vi "Get Index and Type.vi"(8 "error in (no error)":errorcluster, 11 "Tag":string) -> (0 "error out":errorcluster, 2 "Type":T1, 3 "Index":i32)   [LabVIEW 2016, in "CVT.lvlib" / "Current Value Table.lvlib"]
doc: "This VI retrieves a group of indices as defined by the tag names provided. These tags must be retrieved as a single type. If multiple types are requested, error 537165 will be thrown."
uses:
  <vilib>/NI/Current Value Table/Current Value Table.lvlib
  <vilib>/NI/Current Value Table/Type Defs/Data Types.ctl
  <vilib>/NI/Current Value Table/FGVs/Tag Memory Methods.ctl
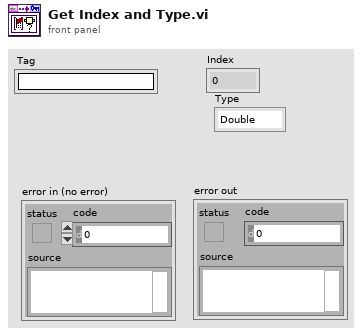
[diagram p1: front panel]
types:
  T1 = typedef "CVT.lvlib/Current Value Table.lvlib/Data Types.ctl" = enum16{"Double", "Single", "I64", "I32", "I16", "I8", "U64", "U32", "U16", "U8", "String", "Boolean", "Array of U8", "Array of U16", "Array of U32", "Array of U64", "Array of I64", "Array of I32", "Array of I16", "Array of I8", "Array of Double", "Array of Single", "Array of Boolean", "Array of String"}
  T2 = typedef "CVT.lvlib/Current Value Table.lvlib/Tag Memory Methods.ctl" = enum16{"Clear", "Read Tag Index", "Read Tag Indices", "Generate Group", "Add Tag", "Overwrite Tag", "Read Description", "Get Stored Tags"}
  T3 = typedef "CVT.lvlib/Current Value Table.lvlib/Tag in Memory.ctl" = cluster{"Index":i32, "Tag":T4}
  T4 = typedef "CVT.lvlib/Current Value Table.lvlib/Single Tag.ctl" = cluster{"Data Type":T1, "Name":string, "Value":string, "Description":string}
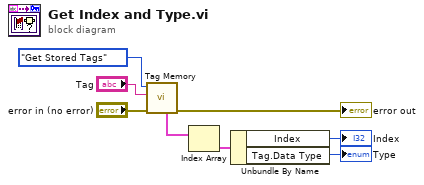
[diagram p0: block diagram]
diagram:
  n1 = call <vilib>:"Tag Memory.vi"("error in (no error)"="error in (no error)", "Tag"="Tag", "Method"=Tag_Memory_Methods."Get Stored Tags") -> ("error out"=→"error out":errorcluster, "Stored Tags"=w5:T3[])  [unwired: 3 in, 4 out]
  n2 = Index Array(array=w5) -> (element=w4:T3)  [unwired: 1 in]
  n3 = Unbundle By Name(w4) -> ("Index"=→"Index":i32, "Tag.Data Type"=→"Type":T1)
